vi "AlertUserMsg1.vi"(10 "Alert":string) -> ()   [LabVIEW 2009]
panel:
  out "length":i32
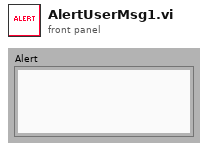
[diagram p1: front panel]
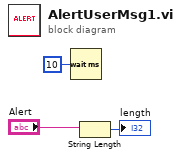
[diagram p0: block diagram]
diagram:
  n1 = Wait (ms)(milliseconds to wait=u32 10) -> ()  [unwired: 1 out]
  n2 = String Length(string="Alert") -> (length=→"length":i32)
